vi "Begin Array.vi"   [LabVIEW 2017, in "LabPack.lvlib" / "Reader.lvclass"]
doc: "Starts reading an array. This must be called before reading and decoding the elements of an array from the MessagePack data."
uses:
  Reader.lvclass
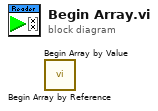
[diagram p0: block diagram]
diagram:
  n1 = call "Begin Array by Reference.vi"() -> ()  [unwired: 9 in, 3 out]
  n2 = call "Begin Array by Value.vi"() -> ()  [unwired: 9 in, 3 out]
